vi "code2str.vi"(2 "错误输入":errorcluster, 3 "input":T1) -> (0 "error out":errorcluster caption="error IO", 1 "output":string)   [LabVIEW 2012]
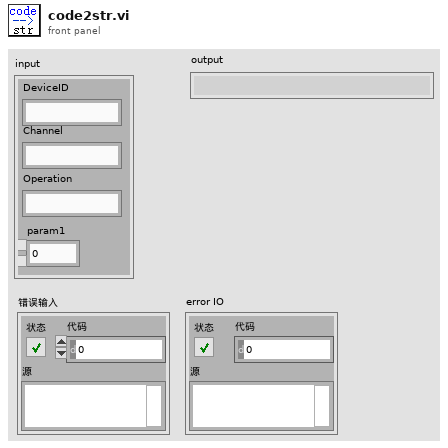
[diagram p1: front panel]
types:
  T1 = cluster{"DeviceID":string, "Channel":string, "param1":dbl, "Operation":string}
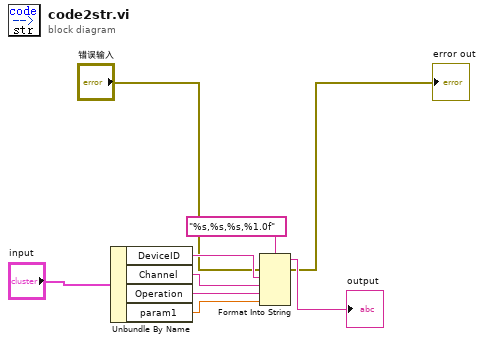
[diagram p0: block diagram]
diagram:
  n1 = Unbundle By Name("input") -> ("DeviceID"=w7:string, "Channel"=w6:string, "Operation"=w5:string, "param1"=w4:dbl)
  n2 = Format Into String(format string="%s,%s,%s,%1.0f" ("格式字符串"), error in="错误输入", w7, w6, w5, w4) -> (resulting string=→"output":string, error out=→"error out":errorcluster)  [unwired: 1 in]
